vi "APX VarianTMP BPP.vi"() -> ()   [LabVIEW 2015]
uses:
  <vilib>/Instr/_visa.llb/VISA Configure Serial Port (Instr).vi
  <userlib>/caLab/Private/Put_DBL-1D_PV-1D.vi
panel:
  out "TMPC5STRSTP 2":string
  in  "APX:AP2Trubo_STOP":bool
  in  "APX:AP2Turbo_START":bool
  out "TMPC5STRSTP":string
  out "SERIAL":string
  out "V-501":refnum<visa-resource-name>="COM4"
  out "APX:AP2TurboF":dbl caption="F_20/Hz"
  out "APX:AP2TurboP":dbl caption="P_20/W"
  out "APX:AP2TurboS":string
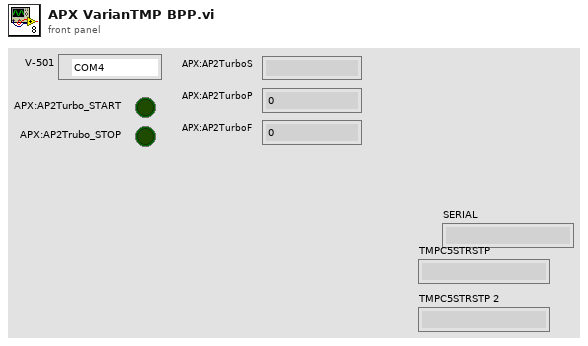
[diagram p1: front panel]
types:
  T1 = enum16{"START", "STOP", "REMOTE/SERIAL", "REMOTE", "SERIAL", "START/STOP", "PUMP STATUS", "Driving Frequency", "PUMP POWER", "PRESSURE"}
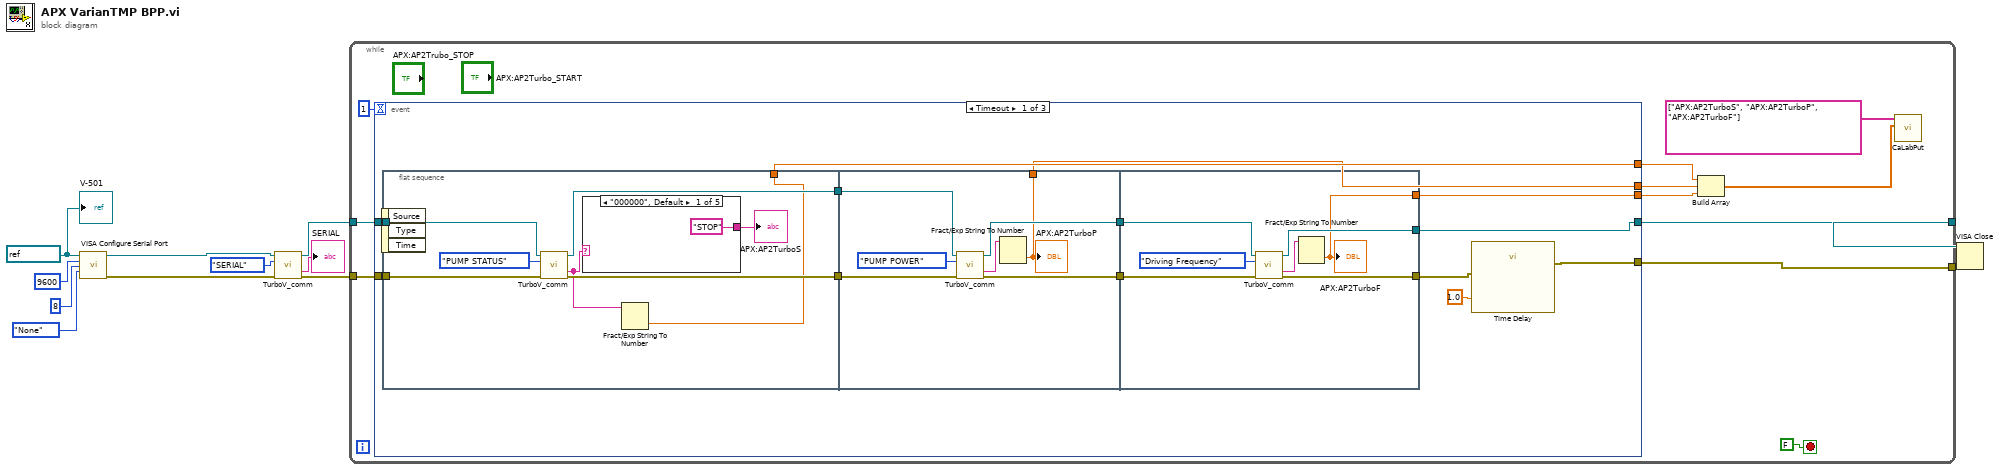
[diagram p0: block diagram]
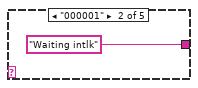
[diagram p2: hidden frame]
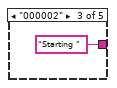
[diagram p3: hidden frame]
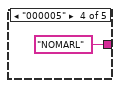
[diagram p4: hidden frame]
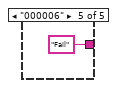
[diagram p5: hidden frame]
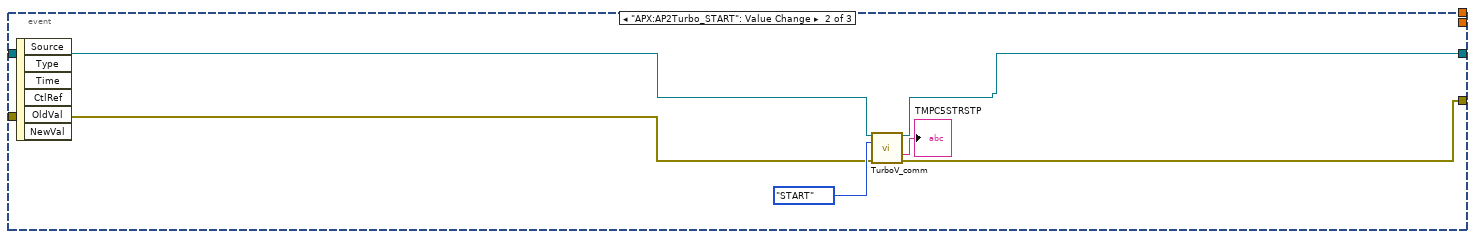
[diagram p6: hidden frame]
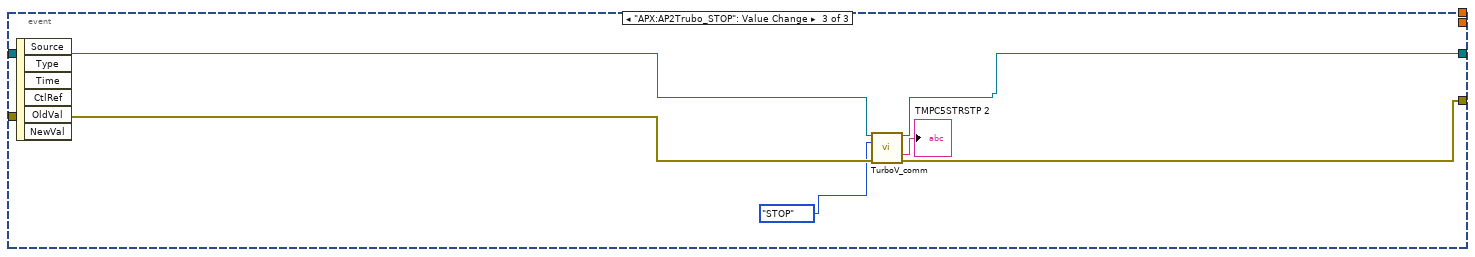
[diagram p7: hidden frame]
diagram:
  w12 = refnum<visa-resource-name> "COM6" ("VISA resource name")
  n1 = call-poly "VISA Configure Serial Port"("VISA resource name"=w12, "baud rate (9600)"=u32 9600, "data bits (8)"=u16 8, "parity (0:none)"=enum16{"None", "Odd", "Even", "Mark", "Space"}."None") -> ("VISA resource name out"=w5:refnum<visa-resource-name>, "error out"=w3:errorcluster)  [unwired: 10 in]
  n2 = call "TurboV_comm.vi"("VISA resource name"=w5, "Command"=T1."SERIAL", "error in (no error)"=w3) -> ("VISA resource name out"=w4:refnum<visa-resource-name>, "read buffer"=→"SERIAL":string, "error out"=w2:errorcluster)  [unwired: 10 in]
  n3 = while {
    tunnel: w4 -> [w23]
    tunnel: w2 -> [w22]
    tunnel: [w21] -> w8
    tunnel: [w19] -> w7
    stop <- FALSE stop-if-true
    n4 = event shown="[0] Timeout" {
      selector: _ -> [_ _ _]
      dyn-events: _ -> [_ _ _]
      timeout: 1 -> [_ _ _]
      tunnel: w23 -> [w32 w65 w72]
      tunnel: w22 -> [w31 w64 w71]
      tunnel: [w27 w67 w74] -> w21
      tunnel: [w28 w66 w73] -> w19
      tunnel: [w26 _ _] -> w16
      tunnel: [w25 _ _] -> w15
      tunnel: [w24 _ _] -> w14
      event Timeout {
        n5 = event-data() -> ()  [unwired: 1 in, 3 out]
        n6 = flat-sequence {
          tunnel: w32 -> [w44]
          tunnel: w31 -> [w43]
          tunnel: [w42] -> w36
          tunnel: [w41] -> w35
          tunnel: [w37] -> w26
          tunnel: w36 -> [w55]
          tunnel: w35 -> [w52]
          tunnel: [w54] -> w34
          tunnel: [w53] -> w33
          tunnel: [w50] -> w25
          tunnel: w34 -> [w63]
          tunnel: w33 -> [w62]
          tunnel: [w59] -> w29
          tunnel: [w58] -> w27
          tunnel: [w57] -> w24
          frame #0 {
            n7 = call "TurboV_comm.vi"("VISA resource name"=w44, "Command"=T1."PUMP STATUS", "error in (no error)"=w43) -> ("VISA resource name out"=w42:refnum<visa-resource-name>, "read buffer"=w38:string, "error out"=w41:errorcluster)  [unwired: 10 in]
            n8 = case shown="\"000000\", Default" w38 {
              tunnel: ["STOP" "Waiting intlk" "Starting " "NOMARL" "Fail"] -> w39
              frame "000000", Default {
              }
              frame "000001" {
              }
              frame "000002" {
              }
              frame "000005" {
              }
              frame "000006" {
              }
            }
            "APX:AP2TurboS" <- w39
            n9 = Fract/Exp String To Number(string=w38) -> (number=w37:dbl)  [unwired: 3 in, 1 out]
          }
          frame #1 {
            n10 = call "TurboV_comm.vi"("VISA resource name"=w55, "Command"=T1."PUMP POWER", "error in (no error)"=w52) -> ("VISA resource name out"=w54:refnum<visa-resource-name>, "read buffer"=w51:string, "error out"=w53:errorcluster)  [unwired: 10 in]
            n11 = Fract/Exp String To Number(string=w51) -> (number=w50:dbl)  [unwired: 3 in, 1 out]
            "APX:AP2TurboP" <- w50
          }
          frame #2 {
            n12 = call "TurboV_comm.vi"("VISA resource name"=w63, "Command"=T1."Driving Frequency", "error in (no error)"=w62) -> ("VISA resource name out"=w58:refnum<visa-resource-name>, "read buffer"=w60:string, "error out"=w59:errorcluster)  [unwired: 10 in]
            n13 = Fract/Exp String To Number(string=w60) -> (number=w57:dbl)  [unwired: 3 in, 1 out]
            "APX:AP2TurboF" <- w57
          }
        }
        n14 = call "Time Delay"("error in (no error)"=w29, "Delay Time (s)"=1.0) -> ("error out"=w28:errorcluster)  [unwired: 9 in]
      }
      event "APX:AP2Turbo_START": Value Change {
        n15 = event-data() -> ()  [unwired: 1 in, 6 out]
        n16 = call "TurboV_comm.vi"("VISA resource name"=w65, "Command"=T1."START", "error in (no error)"=w64) -> ("VISA resource name out"=w67:refnum<visa-resource-name>, "read buffer"=→"TMPC5STRSTP":string, "error out"=w66:errorcluster)  [unwired: 10 in]
      }
      event "APX:AP2Trubo_STOP": Value Change {
        n17 = event-data() -> ()  [unwired: 1 in, 6 out]
        n18 = call "TurboV_comm.vi"("VISA resource name"=w72, "Command"=T1."STOP", "error in (no error)"=w71) -> ("VISA resource name out"=w74:refnum<visa-resource-name>, "read buffer"=→"TMPC5STRSTP 2":string, "error out"=w73:errorcluster)  [unwired: 10 in]
      }
    }
    n19 = Build Array(w16, w15, w14) -> (w13:dbl[])
    n20 = call-poly <userlib>:"CaLabPut.vi"("Values"=w13, "PV Names"=string[] ["APX:AP2TurboS", "APX:AP2TurboP", "APX:AP2TurboF"]) -> ()  [unwired: 6 in, 4 out]
  }
  n21 = VISA Close(VISA resource name=w8, error in (no error)=w7) -> ()  [unwired: 1 out]
  "V-501" <- w12
